vi "LoggingSystem.vi"(8 "stop":bool) -> (0 "Signal2":dbl)   [LabVIEW 2024]
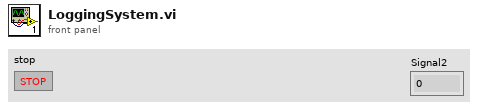
[diagram p1: front panel]
types:
  T1 = cluster{"Devices":refnum<k24>[], "Signals":refnum<k24>[]}
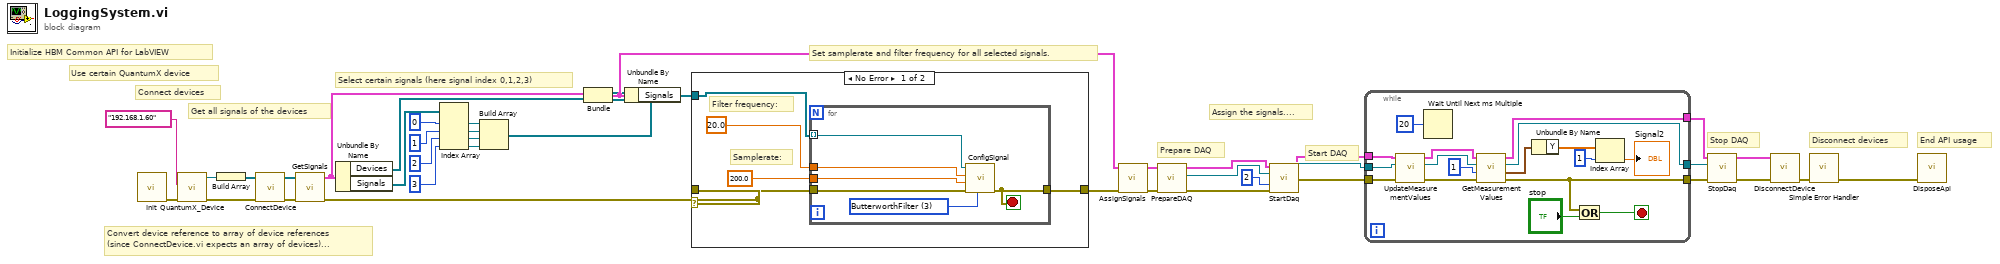
[diagram p0: block diagram]
diagram:
  # "Convert device reference to array of device references\n(since ConnectDevice.vi expects an array of devices)..."
  # "Disconnect devices"
  # "Set samplerate and filter frequency for all selected signals."
  # "Initialize HBM Common API for LabVIEW"
  # "End API usage"
  # "Stop DAQ"
  # "Start DAQ"
  # "Prepare DAQ"
  # "Select certain signals (here signal index 0,1,2,3)"
  # "Get all signals of the devices"
  # "Connect devices"
  # "Use certain QuantumX device"
  # "Assign the signals...."
  n1 = call <userlib>:"Init.vi"() -> ("Error out"=w6:errorcluster)  [unwired: 8 in, 2 out]
  n2 = call <userlib>:"QuantumX_Device.vi"("Error in"=w6, "IPAddress"="192.168.1.60" ("IPAddress of QuantumX device")) -> ("Error out"=w7:errorcluster, "Device"=w4:refnum<k24>)  [unwired: 6 in]
  n3 = Build Array(w4) -> (w3:refnum<k24>[])
  n4 = call <userlib>:"ConnectDevice.vi"("Error in"=w7, "Devices"=w3) -> ("Error out"=w26:errorcluster, "Devices"=w25:refnum<k24>[])  [unwired: 7 in, 1 out]
  n5 = call <userlib>:"GetSignals.vi"("Error in"=w26, "Devices"=w25) -> ("Error out"=w1:errorcluster, "DevicesAndSignals"=w2:T1)  [unwired: 8 in]
  n6 = Unbundle By Name(w2) -> ("Devices"=w17:refnum<k24>[], "Signals"=w21:refnum<k24>[])
  n7 = Index Array(array=w21, index #1=0 ("Index"), index #2=1 ("Index"), index #3=2 ("Index"), index #4=3 ("Index")) -> (element #1=w20:refnum<k24>, element #2=w19:refnum<k24>, element #3=w12:refnum<k24>, element #4=w11:refnum<k24>)
  n8 = Build Array(w20, w19, w12, w11) -> (w18:refnum<k24>[])
  n9 = Bundle(cluster=w2, "Devices"=w17, "Signals"=w18) -> (w23:T1)
  n10 = Unbundle By Name(w23) -> ("Signals"=w39:refnum<k24>[])
  n11 = case shown="No Error" w1 {
    tunnel: w1 -> [w44 w51]
    tunnel: w39 -> [w43 _]
    tunnel: [w42 w51] -> w38
    frame No Error {
      # "Filter frequency:"
      # "Samplerate:"
      n12 = for {
        tunnel: w44 -> [w50]
        tunnel: 200.0 ("SampleRate") -> [w49]
        tunnel: 20.0 ("FilterFrequency") -> [w48]
        tunnel: w43 -> [w47] mode=indexing
        tunnel: [w46] -> w42
        stop <- w46 stop-if-true
        w45 = 3 items=["PresentFilter", "AutoFilter", "BesselFilter", "ButterworthFilter", "HighpassFilter", "LinearPhaseFilter", "NoFilter"] ("FilterType")
        n13 = call <userlib>:"ConfigSignal.vi"("FilterType"=w45, "Error in"=w50, "SampleRate"=w49, "FilterFrequency"=w48, "Signal"=w47) -> ("Error out"=w46:errorcluster)  [unwired: 6 in]
      }
    }
    frame Error {
    }
  }
  n14 = call <userlib>:"AssignSignals.vi"("Error in"=w38, "DevicesAndSignals"=w23) -> ("Error out"=w36:errorcluster, "DevicesAndSignals"=w37:T1)  [unwired: 8 in]
  n15 = call <userlib>:"PrepareDAQ.vi"("Error in"=w36, "DevicesAndSignals"=w37) -> ("Error out"=w33:errorcluster, "DaqMeasurement"=w34:refnum<k24>, "DevicesAndSignals"=w35:T1)  [unwired: 7 in]
  n16 = call <userlib>:"StartDaq.vi"("DevicesAndSignals"=w35, "DaqMeasurement"=w34, "AcquisitionMode"=2, "Error in"=w33) -> ("DevicesAndSignals"=w30:T1, "DaqMeasurement"=w31:refnum<k24>, "Error out"=w32:errorcluster)  [unwired: 7 in, 2 out]
  n17 = while {
    tunnel: w31 -> [w67]
    tunnel: w30 -> [w66]
    tunnel: [w61] -> w28
    tunnel: [w60] -> w27
    tunnel: w32 -> [w68]
    tunnel: [w57] -> w29
    stop <- w58 stop-if-true
    n18 = call <userlib>:"UpdateMeasurementValues.vi"("Error in"=w68, "DaqMeasurement"=w67, "DevicesAndSignals"=w66) -> ("Error out"=w63:errorcluster, "DaqMeasurement"=w64:refnum<k24>, "DevicesAndSignals"=w65:T1)  [unwired: 6 in]
    n19 = Wait Until Next ms Multiple(millisecond multiple=u32 20 ("Vielfache von ms")) -> ()  [unwired: 1 out]
    n20 = call <userlib>:"GetMeasurementValues.vi"("Error in"=w63, "Index"=1 ("Signal index to display"), "DaqMeasurement"=w64, "DevicesAndSignals"=w65) -> ("Error out"=w57:errorcluster, "Waveform"=w56:waveform(dbl), "DaqMeasurement"=w61:refnum<k24>, "DevicesAndSignals"=w60:T1)  [unwired: 2 in, 2 out]
    n21 = Unbundle By Name(w56) -> ("Y"=w55:dbl[])
    n22 = Or(x=w57, y="stop") -> (x .or. y?=w58:bool)
    n23 = Index Array(array=w55, index=1) -> (element=→"Signal2":dbl)
  }
  n24 = call <userlib>:"StopDaq.vi"("Error in"=w29, "DaqMeasurement"=w28, "DevicesAndSignals"=w27) -> ("Error out"=w10:errorcluster, "DevicesAndSignals"=w9:T1)  [unwired: 7 in]
  n25 = call <userlib>:"DisconnectDevice.vi"("Error in"=w10, "DevicesAndSignals"=w9) -> ("Error out"=w8:errorcluster)  [unwired: 9 in]
  n26 = call <vilib>:"Simple Error Handler.vi"("error in (no error)"=w8) -> ("error out"=w24:errorcluster)  [unwired: 4 in, 4 out]
  n27 = call <userlib>:"DisposeApi.vi"("Error in"=w24) -> ()  [unwired: 10 in, 1 out]
